vi "Load Plugin.vi"(8 "error in (no error)":errorcluster, 10 "Plugin":string) -> (0 "error out":errorcluster, 2 "Plugin":refnum<class "Plugin.lvclass">)   [LabVIEW 2020, in "Plugin Loader.lvlib"]
uses:
  Plugin Loader.lvlib
  Plugin/Plugin.lvclass
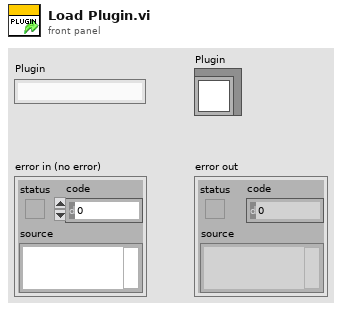
[diagram p1: front panel]
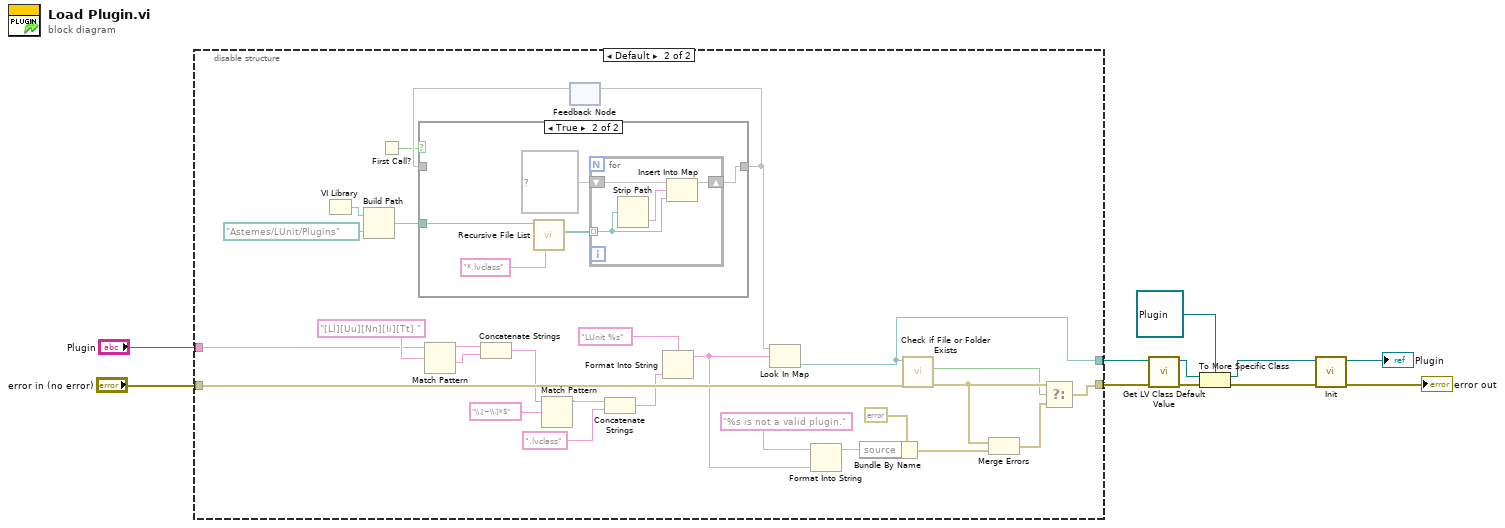
[diagram p0: block diagram]
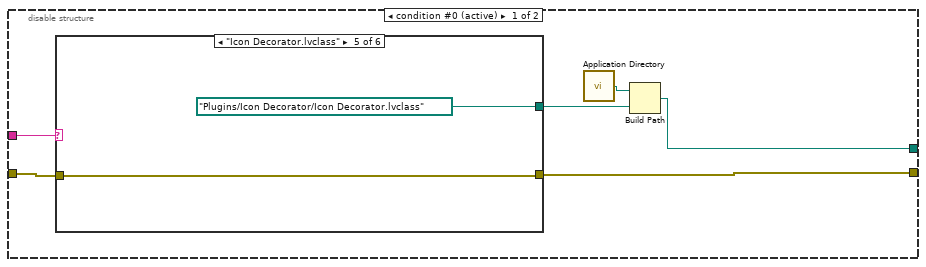
[diagram p2: hidden frame]
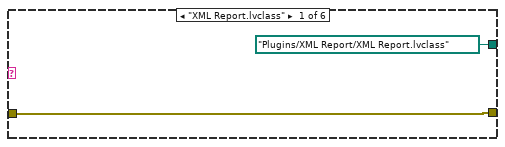
[diagram p3: hidden frame]
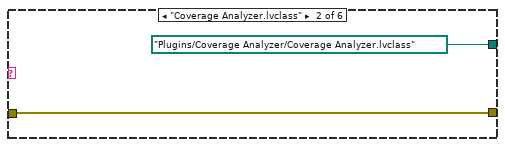
[diagram p4: hidden frame]
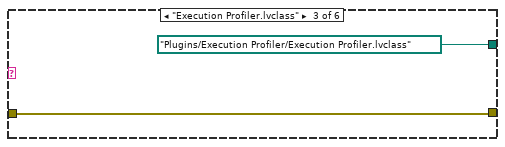
[diagram p5: hidden frame]
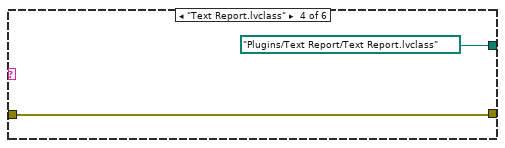
[diagram p6: hidden frame]
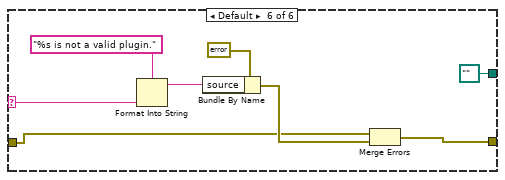
[diagram p7: hidden frame]
diagram:
  n1 = disable-structure shown="Default" {
    disable-tunnel: "Plugin" -> [w17 w49]
    disable-tunnel: "error in (no error)" -> [w16 w61]
    disable-tunnel: [w15 w55] -> w6
    disable-tunnel: [w12 w47] -> w2
    frame condition #0 (active) {
      n2 = case shown="\"Icon Decorator.lvclass\"" w17 {
        selector: w17 -> [_ _ _ _ _ w31]
        tunnel: [w19 w21 w23 w25 w27 w29] -> w15
        tunnel: w16 -> [w19 w21 w23 w25 w27 w28]
        tunnel: [path "Plugins/XML Report/XML Report.lvclass" ("name or relative path") path "Plugins/Coverage Analyzer/Coverage Analyzer.lvclass" ("Relative Path from 1 to 2") path "Plugins/Execution Profiler/Execution Profiler.lvclass" ("Relative Path from 1 to 2") path "Plugins/Text Report/Text Report.lvclass" ("Relative Path from 1 to 2") path "Plugins/Icon Decorator/Icon Decorator.lvclass" ("name or relative path") path "" ("name or relative path")] -> w13
        frame "XML Report.lvclass" {
        }
        frame "Coverage Analyzer.lvclass" {
        }
        frame "Execution Profiler.lvclass" {
        }
        frame "Text Report.lvclass" {
        }
        frame "Icon Decorator.lvclass" {
        }
        frame Default {
          n3 = Format Into String(format string="%s is not a valid plugin.", w31) -> (resulting string=w32:string)  [unwired: 2 in, 1 out]
          n4 = Bundle By Name(cluster=errorcluster {"status"=TRUE, "code"=7, "source"=""} ("error constant"), "source"=w32) -> (w34:errorcluster)
          n5 = Merge Errors(w28, w34) -> (w29:errorcluster)
        }
      }
      n6 = call <vilib>:"Application Directory.vi"() -> ("Application Directory"=w14:path)
      n7 = Build Path(base path=w14, name or relative path=w13) -> (appended path=w12:path)
    }
    frame condition #1 {
      n8 = VI Library() -> (path=w36:path)
      n9 = Build Path(base path=w36, name or relative path=path "Astemes/LUnit/Plugins") -> (appended path=w38:path)
      n10 = First Call?() -> (First Call?: T/F=w39:bool)
      n11 = Match Pattern(string=w49, regular expression="[Ll][Uu][Nn][Ii][Tt] ") -> (before substring=w51:string, after substring=w52:string)  [unwired: 1 in, 2 out]
      n12 = Concatenate Strings(w51, w52) -> (w43:string)
      n13 = Match Pattern(string=w43, regular expression="\\.[~\\.]*$") -> (before substring=w45:string)  [unwired: 1 in, 3 out]
      n14 = feedback #1() -> (w40:map{string, path})  [unwired: 1 in]
      n15 = case shown="True" w39 {
        tunnel: w38 -> [_ w65]
        tunnel: [w63 w64] -> w48
        tunnel: w40 -> [w63 _]
        frame False {
        }
        frame True {
          n16 = call <vilib>:"Recursive File List.vi"("pattern"="*.lvclass", "Folder Path"=w65) -> ("All Files in Dir"=w66:path[])  [unwired: 5 in, 4 out]
          n17 = for {
            shift-right: [w71] -> w64
            shift-left: map{string, path} {} ("map") -> [w72]
            tunnel: w66 -> [w69] mode=indexing
            n18 = Strip Path(path=w69) -> (name=w70:string)  [unwired: 1 out]
            n19 = Insert Into Map(map in=w72, key=w70, value=w69) -> (map out=w71:map{string, path})  [unwired: 2 out]
          }
        }
      }
      n20 = feedback-in #1(w48) -> ()
      n21 = Concatenate Strings(w45, ".lvclass" ("string")) -> (w42:string)
      n22 = Format Into String(format string="LUnit %s" ("Relative Path from 1 to 2"), w42) -> (resulting string=w41:string)  [unwired: 2 in, 1 out]
      n23 = Look In Map(map=w48, key=w41) -> (value=w47:path)  [unwired: 1 in, 1 out]
      n24 = Format Into String(format string="%s is not a valid plugin.", w41) -> (resulting string=w59:string)  [unwired: 2 in, 1 out]
      n25 = Bundle By Name(cluster=errorcluster {"status"=TRUE, "code"=7, "source"=""} ("error constant"), "source"=w59) -> (w60:errorcluster)
      n26 = call <vilib>:"Check if File or Folder Exists.vi"("error in (no error)"=w61, "path"=w47) -> ("error out"=w56:errorcluster, "file or folder exists?"=w54:bool)  [unwired: 7 in, 1 out]
      n27 = Merge Errors(w56, w60) -> (w53:errorcluster)
      n28 = Select(t=w56, s=w54, f=w53) -> (s? t:f=w55:errorcluster)
    }
  }
  n29 = call <vilib>:"Get LV Class Default Value.vi"("error in (no error)"=w6, "class path"=w2) -> ("error out"=w7:errorcluster, "object"=w8:refnum<class>)  [unwired: 8 in]
  n30 = To More Specific Class(target class=refnum<class "Plugin.lvclass"> refnum ("Plugin in"), reference=w8, error in=w7) -> (specific class reference=w4:refnum<class "Plugin.lvclass">, error out=w5:errorcluster)
  n31 = call-dynamic "Init.vi"("error in (no error)"=w5, "Plugin in"=w4) -> ("error out"=→"error out":errorcluster, "Plugin out"=→"Plugin":refnum<class "Plugin.lvclass">)  [unwired: 8 in]
